vi "SP Select Instruments to Use.vi"(10 "Instruments on Station":T1[](array[typedef])) -> (2 "Instrument to Use":T1, 5 "SNA?":bool)   [LabVIEW 2011]
uses:
  server/database/Stations/Instruments/Instrument Record.ctl
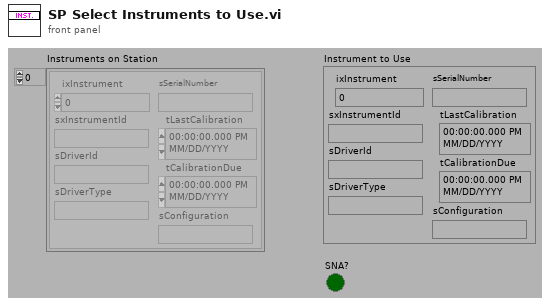
[diagram p1: front panel]
types:
  T1 = typedef "Instrument Record.ctl" = cluster{"ixInstrument":i32, "sxInstrumentId":string, "sDriverId":string, "sDriverType":string, "sSerialNumber":string, "tLastCalibration":timestamp, "tCalibrationDue":timestamp, "sConfiguration":string}
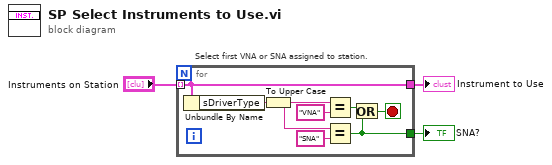
[diagram p0: block diagram]
diagram:
  # "Select first VNA or SNA assigned to station."
  n1 = for {
    tunnel: "Instruments on Station" -> [w9] mode=indexing
    tunnel: [w9] -> w3
    tunnel: [w4] -> w1
    stop <- w5 stop-if-true
    n2 = Unbundle By Name(w9) -> ("sDriverType"=w11:string)
    n3 = To Upper Case(1:w11) -> (0:w7:string)
    n4 = Equal?(x=w7, y="VNA") -> (x = y?=w6:bool)
    n5 = Equal?(x=w7, y="SNA") -> (x = y?=w4:bool)
    n6 = Or(x=w6, y=w4) -> (x .or. y?=w5:bool)
  }
  "Instrument to Use" <- w3
  "SNA?" <- w1
